vi "Map To Driver.vi"(0 "AbstractResourceEnumerator in":refnum<class "AbstractResourceEnumerator.lvclass">, 5 "Driver Name":string, 11 "error in (no error)":errorcluster) -> (4 "AbstractResourceEnumerator out":refnum<class "AbstractResourceEnumerator.lvclass">, 6 "Driver":refnum<class "Driver.lvclass">, 15 "error out":errorcluster)   [LabVIEW 2023, in "HAF.lvlib" / "AbstractResourceEnumerator.lvclass"]
doc: "Passed an alias or canonical name it returns a concrete Driver (Instrument) instance or raises error 200 if no match found."
uses:
  AbstractResourceEnumerator.lvclass
  Driver/Driver.lvclass
  AbstractResourceEnumerator.lvclass/AbstractResourceEnumerator.ctl
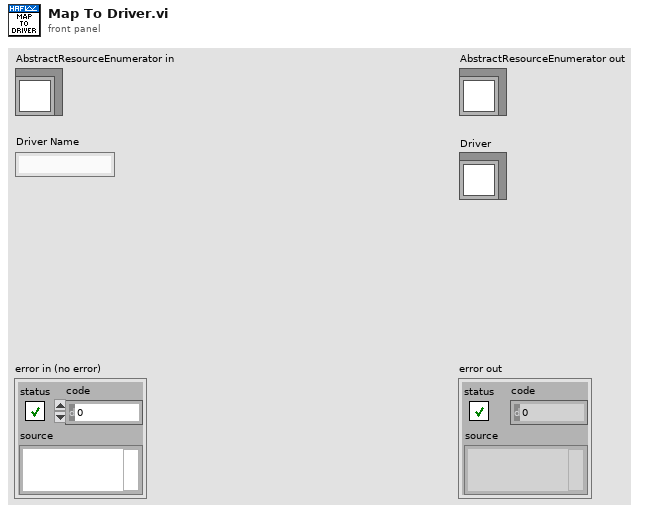
[diagram p1: front panel]
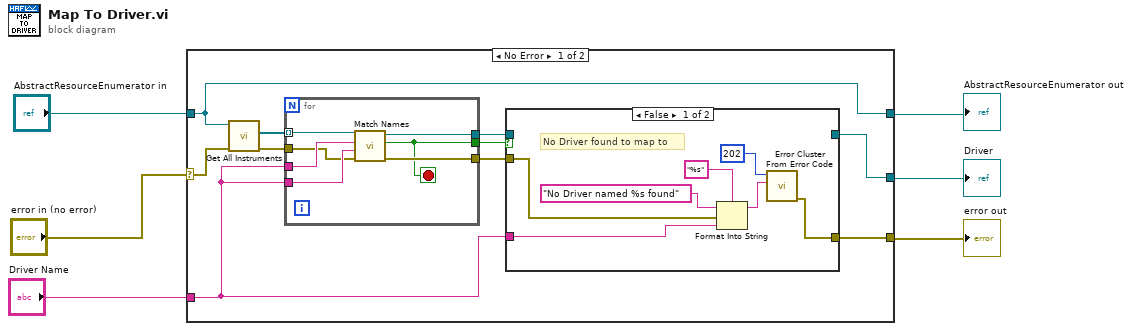
[diagram p0: block diagram]
diagram:
  n1 = case shown="No Error" "error in (no error)" {
    selector: "error in (no error)" -> [w14 w33]
    tunnel: "AbstractResourceEnumerator in" -> [w7 w34]
    tunnel: [w7 w34] -> w3
    tunnel: [w9 w33] -> w1
    tunnel: "Driver Name" -> [w8 _]
    tunnel: [w10 _] -> w2
    frame No Error {
      n2 = call-dynamic "Get All Instruments.vi"("error in (no error)"=w14, "AbstractResourceEnumerator in"=w7) -> ("error out"=w15:errorcluster, "Instruments"=w16:refnum<class "Driver.lvclass">[])  [unwired: 7 in, 1 out]
      n3 = for {
        tunnel: w16 -> [w32] mode=indexing
        tunnel: w8 -> [w31]
        tunnel: w8 -> [w30]
        tunnel: w15 -> [w29]
        tunnel: [w28] -> w12
        tunnel: [w27] -> w11
        tunnel: [w26] -> w13
        stop <- w26 stop-if-true
        n4 = call-dynamic "Match Names.vi"("error in (no error)"=w29, "Canonical"=w30, "Alias"=w31, "Driver in"=w32) -> ("error out"=w27:errorcluster, "Recognised"=w26:bool, "Driver out"=w28:refnum<class "Driver.lvclass">)  [unwired: 5 in]
      }
      n5 = case shown="False" w13 {
        tunnel: w12 -> [_ w25]
        tunnel: w11 -> [w21 w24]
        tunnel: [_ w25] -> w10
        tunnel: [w17 w24] -> w9
        tunnel: w8 -> [w18 _]
        frame False {
          # "No Driver found to map to"
          n6 = Format Into String(format string="%s", initial string="No Driver named %s found", error in=w21, w18) -> (resulting string=w22:string)  [unwired: 1 out]
          n7 = call <vilib>:"Error Cluster From Error Code.vi"("error message (\"\")"=w22, "error code (0)"=202) -> ("error out"=w17:errorcluster)  [unwired: 7 in]
        }
        frame True {
          # "Found a Driver that mapped to the passed name"
        }
      }
    }
    frame Error {
    }
  }
  "error out" <- w1
  "AbstractResourceEnumerator out" <- w3
  "Driver" <- w2
